vi "getClaseDB.vi"(8 "error in":errorcluster, 11 "claseDB.lvclass":refnum<class "claseDB.lvclass">) -> (0 "error out":errorcluster, 2 "datosClaseDB":T1, 3 "claseDB.lvclass 2":refnum<class "claseDB.lvclass">)   [LabVIEW 2014, in "claseDB.lvclass"]
uses:
  claseDB.lvclass
  claseDB.lvclass/claseDB.ctl
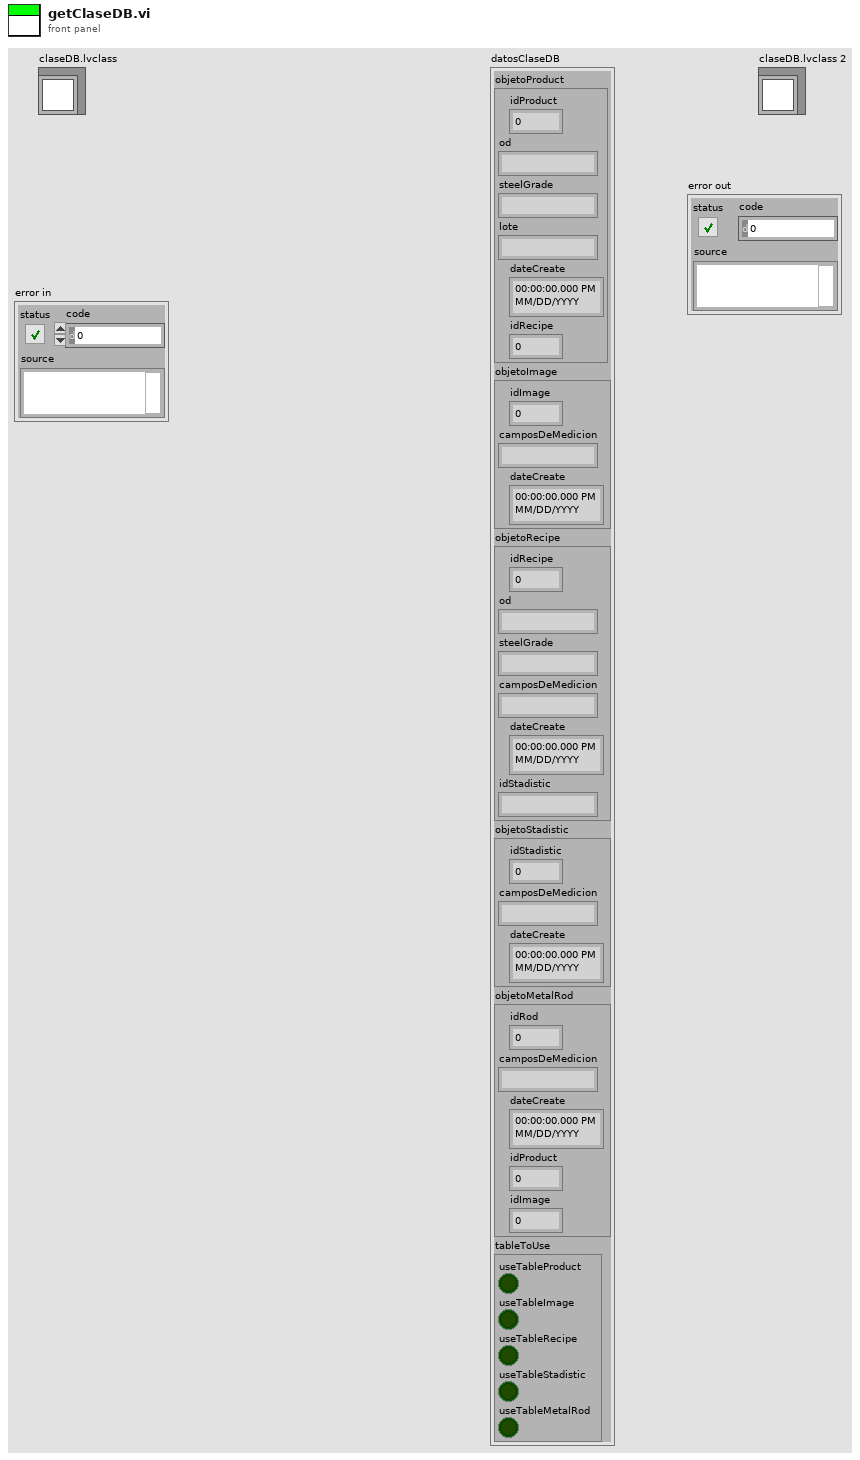
[diagram p1: front panel]
types:
  T1 = cluster{"objetoProduct":cluster{"idProduct":dbl, "od":string, "steelGrade":string, "lote":string, "dateCreate":timestamp, "idRecipe":dbl}, "objetoImage":cluster{"idImage":dbl, "camposDeMedicion":string, "dateCreate":timestamp}, "objetoRecipe":cluster{"idRecipe":dbl, "od":string, "steelGrade":string, "camposDeMedicion":string, "dateCreate":timestamp, "idStadistic":string}, "objetoStadistic":cluster{"idStadistic":dbl, "camposDeMedicion":string, "dateCreate":timestamp}, "objetoMetalRod":cluster{"idRod":dbl, "camposDeMedicion":string, "dateCreate":timestamp, "idProduct":dbl, "idImage":dbl}, "tableToUse":cluster{"useTableProduct":bool, "useTableImage":bool, "useTableRecipe":bool, "useTableStadistic":bool, "useTableMetalRod":bool}}
  T2 = cluster{"idProduct":dbl, "od":string, "steelGrade":string, "lote":string, "dateCreate":timestamp, "idRecipe":dbl}
  T3 = cluster{"idImage":dbl, "camposDeMedicion":string, "dateCreate":timestamp}
  T4 = cluster{"idRecipe":dbl, "od":string, "steelGrade":string, "camposDeMedicion":string, "dateCreate":timestamp, "idStadistic":string}
  T5 = cluster{"idStadistic":dbl, "camposDeMedicion":string, "dateCreate":timestamp}
  T6 = cluster{"idRod":dbl, "camposDeMedicion":string, "dateCreate":timestamp, "idProduct":dbl, "idImage":dbl}
  T7 = cluster{"useTableProduct":bool, "useTableImage":bool, "useTableRecipe":bool, "useTableStadistic":bool, "useTableMetalRod":bool}
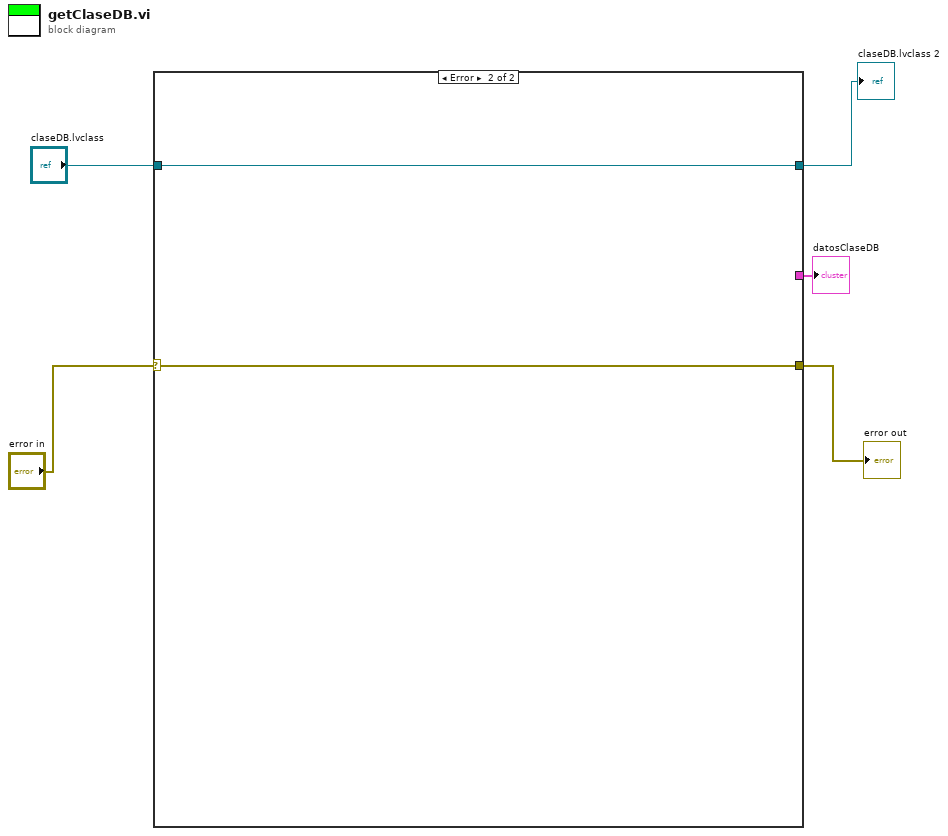
[diagram p0: block diagram]
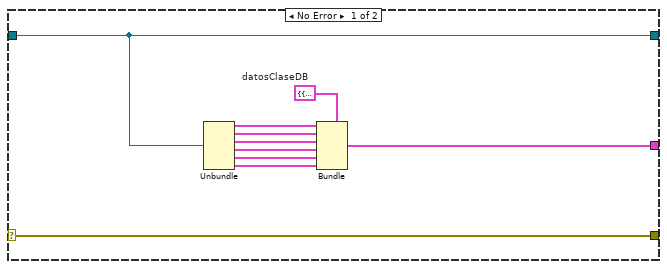
[diagram p2: hidden frame]
diagram:
  n1 = case shown="Error" "error in" {
    selector: "error in" -> [w7 w17]
    tunnel: "claseDB.lvclass" -> [w6 w16]
    tunnel: [w8 _] -> w3
    tunnel: [w7 w17] -> w2
    tunnel: [w6 w16] -> w1
    frame No Error {
      w9 = T1 {"objetoProduct"={"idProduct"=0.0, "od"="", "steelGrade"="", "lote"="", "dateCreate"=timestamp(0 s since 1904-01-01), "idRecipe"=0.0}, "objetoImage"={"idImage"=0.0, "camposDeMedicion"="", "dateCreate"=timestamp(0 s since 1904-01-01)}, "objetoRecipe"={"idRecipe"=0.0, "od"="", "steelGrade"="", "camposDeMedicion"="", "dateCreate"=timestamp(0 s since 1904-01-01), "idStadistic"=""}, "objetoStadistic"={"idStadistic"=0.0, "camposDeMedicion"="", "dateCreate"=timestamp(0 s since 1904-01-01)}, "objetoMetalRod"={"idRod"=0.0, "camposDeMedicion"="", "dateCreate"=timestamp(0 s since 1904-01-01), "idProduct"=0.0, "idImage"=0.0}, "tableToUse"={"useTableProduct"=FALSE, "useTableImage"=FALSE, "useTableRecipe"=FALSE, "useTableStadistic"=FALSE, "useTableMetalRod"=FALSE}}  # datosClaseDB
      n2 = Unbundle(w6) -> (w15:T2, w14:T3, w13:T4, w12:T5, w11:T6, w10:T7)
      n3 = Bundle(cluster=w9, "objetoProduct"=w15, "objetoImage"=w14, "objetoRecipe"=w13, "objetoStadistic"=w12, "objetoMetalRod"=w11, "tableToUse"=w10) -> (w8:T1)
    }
    frame Error {
    }
  }
  "error out" <- w2
  "datosClaseDB" <- w3
  "claseDB.lvclass 2" <- w1
